vi "abouttest.vi"   [LabVIEW 2015]
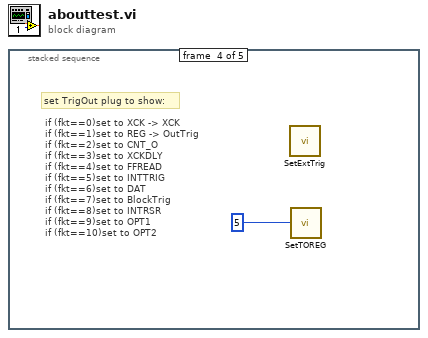
[diagram p0: block diagram]
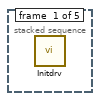
[diagram p2: hidden frame]
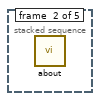
[diagram p3: hidden frame]
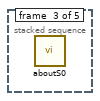
[diagram p4: hidden frame]
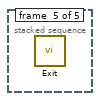
[diagram p5: hidden frame]
diagram:
  n1 = stacked-sequence {
    frame #0 {
      n2 = call "Initdrv.vi"() -> ()  [unwired: 1 in]
    }
    frame #1 {
      n3 = call "about.vi"() -> ()  [unwired: 1 in]
    }
    frame #2 {
      n4 = call "aboutS0.vi"() -> ()  [unwired: 1 in]
    }
    frame #3 {
      # "set TrigOut plug to show:"
      # "if (fkt==0)set to XCK -> XCK\nif (fkt==1)set to REG -> OutTrig\nif (fkt==2)set to CNT_O\nif (fkt==3)set to XCKDLY\nif (fkt==4)set to FFREAD\nif (fkt==5)set to INTTRIG\nif (fkt==6)set to DAT\nif (fkt==7)set to BlockTrig\nif (fkt==8)set to INTRSR\nif (fkt==9)set to OPT1\nif (fkt==10)set to OPT2"
      n5 = call "SetExtTrig.vi"() -> ()  [unwired: 1 in]
      n6 = call "SetTOREG.vi"("fkt"=u8 5) -> ()
    }
    frame #4 {
      n7 = call "Exit.vi"() -> ()  [unwired: 1 in]
    }
  }
